vi "Speed TRA test.vi"() -> ()   [LabVIEW 2019]
uses:
  <vilib>/Platform/TimedLoop/XDataNode/timing_clust.ctl
  <vilib>/Platform/TimedLoop/XDataNode/nitl_modes.ctl
  <vilib>/Platform/TimedLoop/XDataNode/wakeup.ctl
  <vilib>/platform/TimedLoop/XDataNode/XDataNode.xnode
  <vilib>/Platform/TimedLoop/XDataNode/XDNodeRunTimeDep.lvlib
panel:
  in  "stop":bool
  out "second":dbl
  out "complet?":bool
  in  "t2":dbl format="%#_13g"
  out "Waveform Chart":dbl(graph)
  in  "dt(s)":dbl
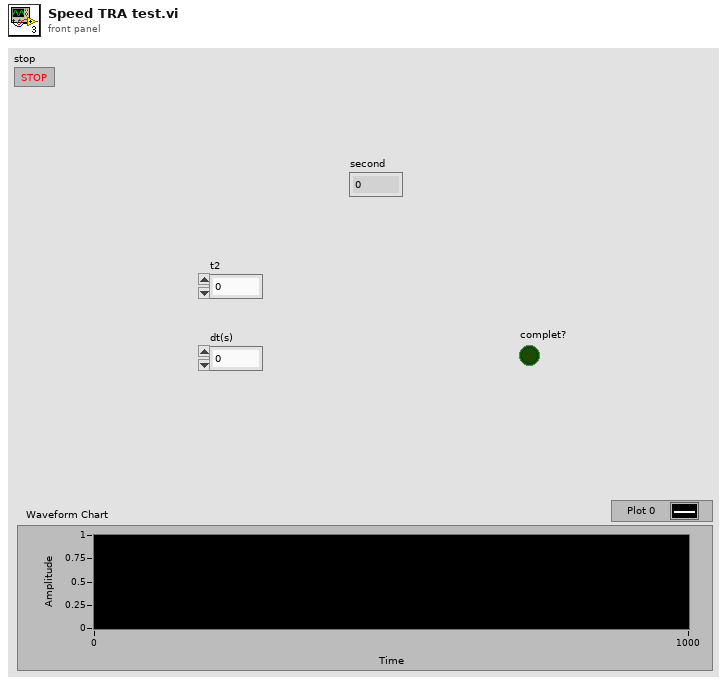
[diagram p1: front panel]
types:
  T1 = typedef "XDNodeRunTimeDep.lvlib/timing_clust.ctl" = cluster{"Expected End [f-1]":u64, "Actual End [f-1]":u64, "Finished Late? [f-1]":bool, "Expected End [i-1]":u64, "Actual End [i-1]":u64, "Finished Late? [i-1]":bool, "Expected Start [i]":u64, "Actual Start [i]":u64, "Expected Start [f]":u64, "Actual Start [f]":u64, "Source Name":string, "Structure Name":string, "Period":i64, "Deadline":i64, "Offset":i64, "Start":i64, "Priority":i32, "Timeout":i32, "Mode":T2, "Wakeup Reason":T3, "Error":errorcluster, "Source Type":string, "Secondary Source Type":string, "Global End Time":u64, "Global Start Time":u64, "Frame Duration":u64, "Iteration Duration":u64, "Assigned CPU":i32, "I/O Scan Engine Mode":u32}
  T2 = typedef "XDNodeRunTimeDep.lvlib/nitl_modes.ctl" = enum32{"No Change", "Process missed periods, maintain original phase", "Discard missed periods, maintain original phase", "Process missed periods, ignore original phase", "Discard missed periods, ignore original phase"}
  T3 = typedef "XDNodeRunTimeDep.lvlib/wakeup.ctl" = enum32{"Normal", "Aborted", "Asynchronous wakeup", "Timing source error", "Timed loop error", "Timeout"}
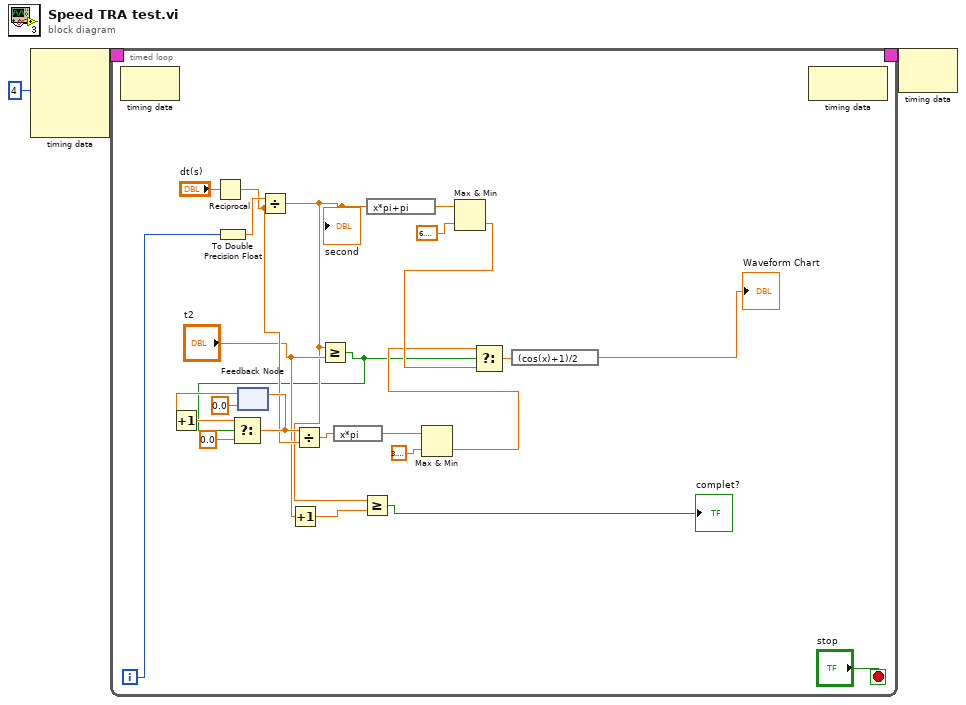
[diagram p0: block diagram]
diagram:
  n1 = node-c288(i64 4 ("Period")) -> (w3:T1)  [unwired: 3 in]
  n2 = timed-loop {
    timing: w3 -> [_]
    timing-out: [_] -> w2
    i -> [w5]
    stop <- "stop" stop-if-true
    n3 = node-c288() -> ()  [unwired: 1 in, 1 out]
    n4 = Reciprocal(x="dt(s)") -> (1/x=w16:dbl)
    n5 = To Double Precision Float(number=w5) -> (double precision float=w26:dbl)
    n6 = feedback #1(0.0 ("f")) -> (w20:dbl)
    n7 = Increment(x=w20) -> (x+1=w18:dbl)
    n8 = Divide(x=w26, y=w16) -> (x/y=w8:dbl)
    "second" <- w8
    n9 = Increment(x="t2") -> (x+1=w9:dbl)
    n10 = Greater Or Equal?(x=w8, y="t2") -> (x >= y?=w7:bool)
    n11 = Select(t=w18, s=w7, f=0.0) -> (s? t:f=w17:dbl)
    n12 = feedback-in #1(w17) -> ()
    n13 = Divide(x=w17, y=w16) -> (x/y=w15:dbl)
    n14 = expression code="x*pi"(w15) -> (w14:dbl)
    n15 = Greater Or Equal?(x=w8, y=w9) -> (x >= y?=→"complet?":bool)
    n16 = expression code="x*pi+pi"(w8) -> (w25:dbl)
    n17 = Max & Min(x=w14, y=3.141592653589793) -> (min(x,y)=w12:dbl)  [unwired: 1 out]
    n18 = Max & Min(x=w25, y=6.283185307179586) -> (min(x,y)=w23:dbl)  [unwired: 1 out]
    n19 = Select(t=w12, s=w7, f=w23) -> (s? t:f=w22:dbl)
    n20 = expression code="(cos(x)+1)/2"(w22) -> (→"Waveform Chart":dbl)
    n21 = node-c288() -> ()  [unwired: 1 in, 1 out]
  }
  n22 = node-c288(w2) -> ()  [unwired: 1 out]
